vi "loadTDMS.vi"(8 "错误输入（无错误）":errorcluster) -> (0 "错误输出":errorcluster, 1 "file path out":path, 2 "数据":waveform(dbl)[](array[waveform]), 3 "输出簇":T1)   [LabVIEW 2013]
uses:
  <vilib>/Utility/error.llb/Error Cluster From Error Code.vi
  <vilib>/ErrorRing/Error Ring.xnode
panel:
  in  "取消按钮":bool
  in  "确定按钮":bool
  in  "Choose *.tdms file":path
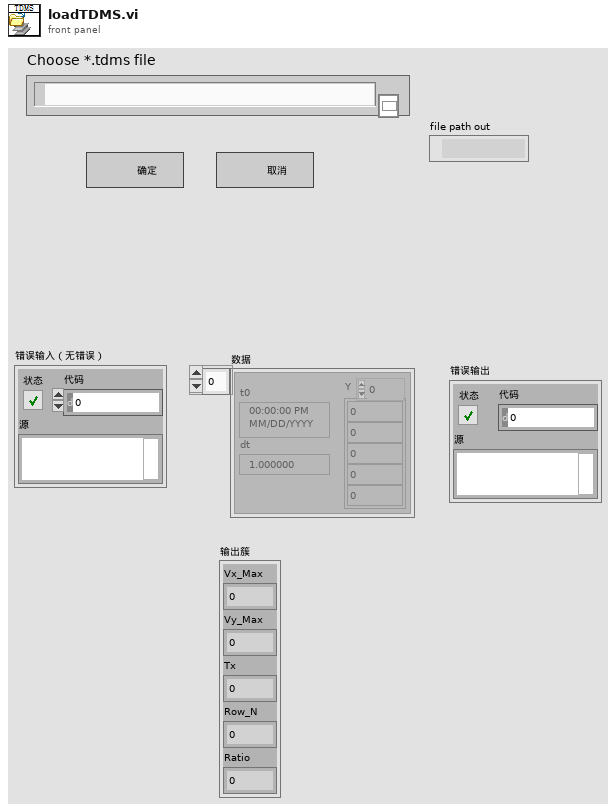
[diagram p1: front panel]
types:
  T1 = cluster{"Vx_Max":dbl, "Vy_Max":dbl, "Tx":dbl, "Row_N":i32, "Ratio":dbl}
  T2 = cluster{"[0]":dbl, "[1]":dbl, "[2]":dbl, "[3]":dbl, "[4]":dbl, "[5]":dbl, "[6]":dbl, "[7]":dbl, "[8]":dbl}
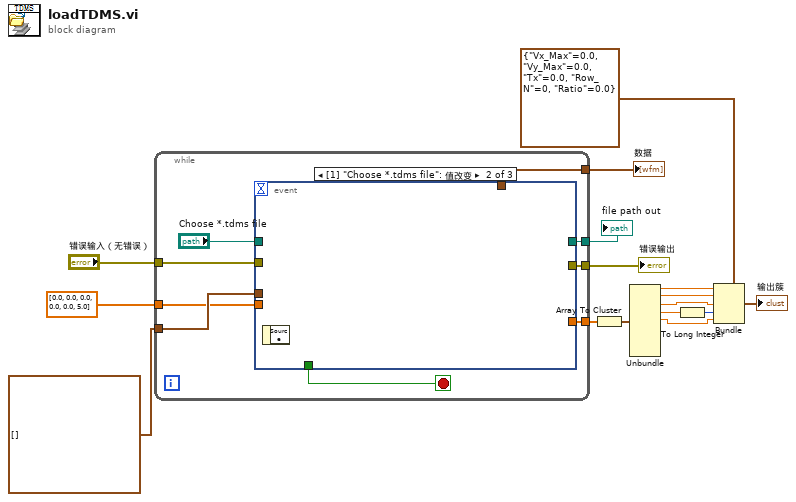
[diagram p0: block diagram]
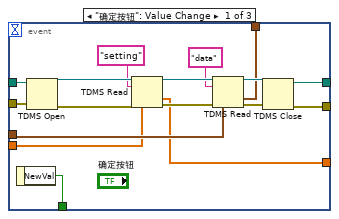
[diagram p2: hidden frame]
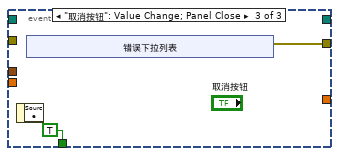
[diagram p3: hidden frame]
diagram:
  n1 = while {
    tunnel: "错误输入（无错误）" -> [w24]
    tunnel: waveform(dbl)[] [] -> [w23]
    tunnel: [w22] -> w14
    tunnel: [w21] -> w13
    tunnel: dbl[] [0.0, 0.0, 0.0, 0.0, 0.0, 5.0] -> [w19]
    tunnel: [w18] -> w11
    tunnel: [w17] -> w1
    stop <- w20 stop-if-true
    n2 = event shown="[1] \"Choose *.tdms file\": 值改变" {
      selector: _ -> [_ _ _]
      dyn-events: _ -> [_ _ _]
      timeout: _ -> [_ _ _]
      tunnel: "Choose *.tdms file" -> [w42 _ _]
      tunnel: w24 -> [w41 _ _]
      tunnel: w23 -> [w38 _ _]
      tunnel: [w37 _ _] -> w22
      tunnel: [w36 _ w43] -> w21
      tunnel: [w35 _ TRUE] -> w20
      tunnel: w19 -> [w29 _ _]
      tunnel: [w27 _ _] -> w18
      tunnel: [w26 _ _] -> w17
      event "确定按钮": Value Change {
        n3 = event-data() -> ("NewVal"=w35:bool)  [unwired: 1 in]
        n4 = TDMS Open(8:w41, 11:w42) -> (0:w34:errorcluster, 3:w31:refnum<k34>)  [unwired: 5 in]
        n5 = TDMS Read(0:w31, 5:"setting" ("组名称输入"), 11:w34, 12:w29) -> (4:w32:refnum<k34>, 10:w27:dbl[], 15:w33:errorcluster)  [unwired: 4 in, 3 out]
        n6 = TDMS Read(0:w32, 5:"data" ("组名称输入"), 11:w33, 12:w38) -> (4:w40:refnum<k34>, 10:w37:waveform(dbl)[], 15:w39:errorcluster)  [unwired: 4 in, 3 out]
        n7 = TDMS Close(8:w39, 11:w40) -> (0:w36:errorcluster, 3:w26:path)
      }
      event "Choose *.tdms file": Value Change {
        n8 = event-data() -> ()  [unwired: 1 in, 1 out]
      }
      event "取消按钮": Value Change; Panel Close {
        n9 = event-data() -> ()  [unwired: 1 in, 1 out]
        n10 = xnode "错误下拉列表"() -> ("错误输出"=w43:errorcluster)
      }
    }
  }
  "数据" <- w14
  "错误输出" <- w13
  "file path out" <- w1
  n11 = Array To Cluster(array=w11) -> (cluster=w7:T2)
  n12 = Unbundle(w7) -> ("[0]"=w5:dbl, "[1]"=w4:dbl, "[2]"=w3:dbl, "[3]"=w6:dbl, "[4]"=w2:dbl)  [unwired: 4 out]
  n13 = To Long Integer(number=w6) -> (32bit integer=w10:i32)
  n14 = Bundle(cluster=T1 {"Vx_Max"=0.0, "Vy_Max"=0.0, "Tx"=0.0, "Row_N"=0, "Ratio"=0.0}, "Vx_Max"=w5, "Vy_Max"=w4, "Tx"=w3, "Row_N"=w10, "Ratio"=w2) -> (→"输出簇":T1)
